vi "RidgeCV.vi"(8 "error in":errorcluster) -> (0 "error out":errorcluster, 3 "out":refnum<class "RidgeCV.lvclass">)   [LabVIEW 2020]
doc: "Ridge regression with built-in cross-validation.\n\n See glossary entry for :term:`cross-validation estimator`.\n\n By default, it performs efficient Leave-One-Out Cross-Validation.\n\n Read more in the :ref:`User Guide <ridge_regression>`.\n\n Parameters\n ----------\n alphas : ndarray of shape (n_alphas,), default=(0.1, 1.0, 10.0)\n Array of alpha values to try.\n Regularization strength; must be a positive float. Regularization\n improves the conditioning of the problem and reduces the variance of\n the estimates. Larger values specify stronger regularization.\n Alpha corresponds to ``1 / (2C)`` in other linear models such as\n :class:`~sklearn.linear_model.LogisticRegression` or\n :class:`~sklearn.svm.LinearSVC`.\n If using Leave-One-Out cross-validation, alphas must be positive.\n\n fit_intercept : bool, default=True\n Whether to calculate the intercept for this model. If set\n to false, no intercept will be used in calculations\n (i.e. data is expected to be centered).\n\n normalize : bool, default=False\n This parameter is ignored when ``fit_intercept`` is set to False.\n If True, the regressors X will be normalized before regression by\n subtracting the mean and dividing by the l2-norm.\n If you wish to standardize, please use\n :class:`~sklearn.preprocessing.StandardScaler` before calling ``fit``\n on an estimator with ``normalize=False``.\n\n scoring : string, callable, default=None\n A string (see model evaluation documentation) or\n a scorer callable object / function with signature\n ``scorer(estimator, X, y)``.\n If None, the negative mean squared error if cv is 'auto' or None\n (i.e. when using leave-one-out cross-validation), and r2 score\n otherwise.\n\n cv : int, cross-validation generator or an iterable, default=None\n Determines the cross-validation splitting strategy.\n Possible inputs for cv are:\n\n - None, to use the efficient Leave-One-Out cross-validation\n - integer, to specify the number of folds.\n - :term:`CV splitter`,\n - An iterable yielding (train, test) splits as arrays of indices.\n\n For integer/None inputs, if ``y`` is binary or multiclass,\n :class:`~sklearn.model_selection.StratifiedKFold` is used, else,\n :class:`~sklearn.model_selection.KFold` is used.\n\n Refer :ref:`User Guide <cross_validation>` for the various\n cross-validation strategies that can be used here.\n\n gcv_mode : {'auto', 'svd', eigen'}, default='auto'\n Flag indicating which strategy to use when performing\n Leave-One-Out Cross-Validation. Options are::\n\n 'auto' : use 'svd' if n_samples > n_features, otherwise use 'eigen'\n 'svd' : force use of singular value decomposition of X when X is\n dense, eigenvalue decomposition of X^T.X when X is sparse.\n 'eigen' : force computation via eigendecomposition of X.X^T\n\n The 'auto' mode is the default and is intended to pick the cheaper\n option of the two depending on the shape of the training data.\n\n store_cv_values : bool, default=False\n Flag indicating if the cross-validation values corresponding to\n each alpha should be stored in the ``cv_values_`` attribute (see\n below). This flag is only compatible with ``cv=None`` (i.e. using\n Leave-One-Out Cross-Validation).\n\n alpha_per_target : bool, default=False\n Flag indicating whether to optimize the alpha value (picked from the\n `alphas` parameter list) for each target separately (for multi-output\n settings: multiple prediction targets). When set to `True`, after\n fitting, the `alpha_` attribute will contain a value for each target.\n When set to `False`, a single alpha is used for all targets.\n\n .. versionadded:: 0.24\n\n Attributes\n ----------\n cv_values_ : ndarray of shape (n_samples, n_alphas) or shape (n_samples, n_targets, n_alphas), optional\n Cross-validation values for each alpha (only available if\n ``store_cv_values=True`` and ``cv=None``). After ``fit()`` has been\n called, this attribute will contain the mean squared errors\n (by default) or the values of the ``{loss,score}_func`` function\n (if provided in the constructor).\n\n coef_ : ndarray of shape (n_features) or (n_targets, n_features)\n Weight vector(s).\n\n intercept_ : float or ndarray of shape (n_targets,)\n Independent term in decision function. Set to 0.0 if\n ``fit_intercept = False``.\n\n alpha_ : float or ndarray of shape (n_targets,)\n Estimated regularization parameter, or, if ``alpha_per_target=True``,\n the estimated regularization parameter for each target.\n\n best_score_ : float or ndarray of shape (n_targets,)\n Score of base estimator with best alpha, or, if\n ``alpha_per_target=True``, a score for each target.\n\n .. versionadded:: 0.23\n\n \nAvailable methods:\nGet Attributes\nGet Params\nSet Params"
uses:
  RidgeCV.lvclass
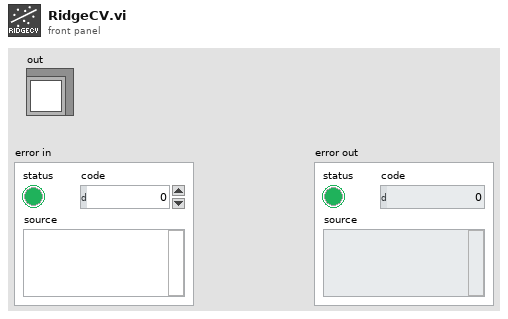
[diagram p1: front panel]
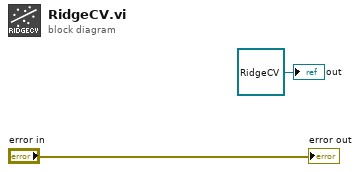
[diagram p0: block diagram]
diagram:
  "out" <- refnum<class "RidgeCV.lvclass"> refnum ("model")
  "error out" <- "error in"
